vi "Open File Offline.vi"(8 "error in (no error)":errorcluster, 11 "File Path":path) -> (0 "error out":errorcluster, 3 "pcap reference":u64)   [LabVIEW 2025, in "Automotive Ethernet Bus Monitor UI.lvlib" / "lvwpcap.lvlib"]
uses:
  lvwpcap.lvlib
  lvwpcap.dll
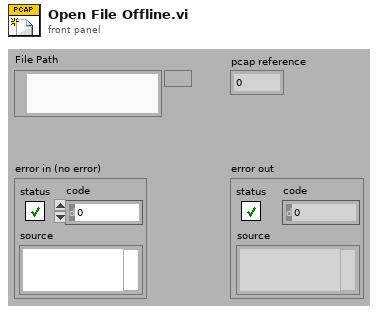
[diagram p1: front panel]
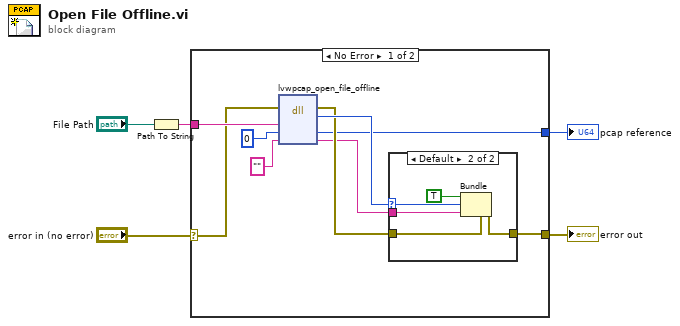
[diagram p0: block diagram]
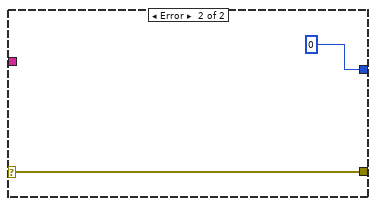
[diagram p3: hidden frame]
diagram:
  n1 = Path To String(path="File Path") -> (string=w3:string)
  n2 = case shown="No Error" "error in (no error)" {
    selector: "error in (no error)" -> [w12 w22]
    tunnel: [w10 w22] -> w5
    tunnel: [w9 u64 0 ("pcap")] -> w1
    tunnel: w3 -> [w14 _]
    frame No Error {
      n3 = dll-call lib="lvwpcap.dll" fn="lvwpcap_open_file_offline"(error in=w12, "file_path"=w14, "pcap"=u64 0, "error_string"="") -> (error out=w11:errorcluster, "return type"=w13:u64, "pcap"=w9:u64, "error_string"=w8:string)  [unwired: 3 in, 1 out]
      n4 = case shown="Default" w13 {
        selector: w13 -> [_ w19]
        tunnel: w8 -> [_ w18]
        tunnel: w11 -> [w15 w20]
        tunnel: [w15 w16] -> w10
        frame 0 {
        }
        frame Default {
          n5 = Bundle(cluster=w20, "status"=TRUE, "code"=w19, "source"=w18) -> (w16:errorcluster)
        }
      }
    }
    frame Error {
    }
  }
  "error out" <- w5
  "pcap reference" <- w1
